vi "Name Bundle Selection.vi"(9 "Current Loop Iteration Even":bool, 10 "Bundler Selections":cluster{string[]}[](array[cluster]), 11 "Node Number":string) -> (2 "Appended Bundler Selections":cluster{string[]}[](array[cluster]))   [LabVIEW 2014, in "Initialization and IO Node Scripting.lvlib"]
uses:
  Initialization and IO Node Scripting.lvlib
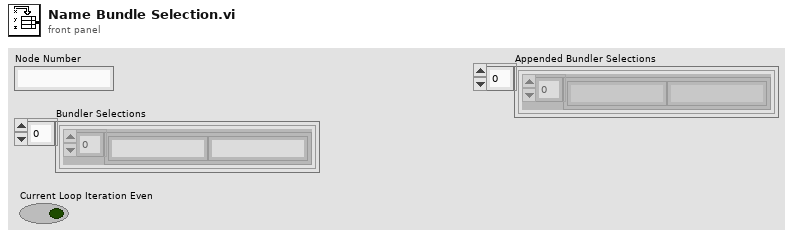
[diagram p1: front panel]
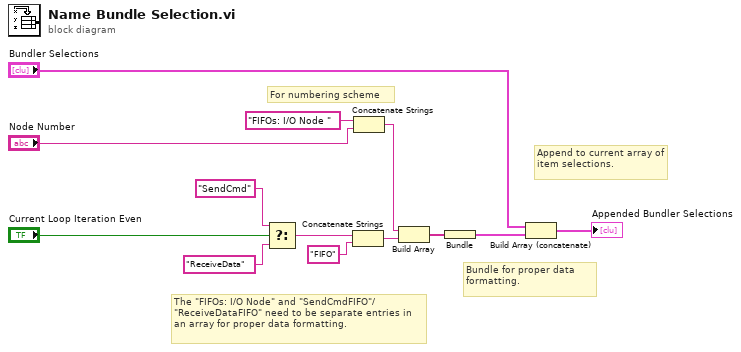
[diagram p0: block diagram]
diagram:
  # "Append to current array of item selections."
  # "Bundle for proper data formatting."
  # "For numbering scheme"
  # "The \"FIFOs: I/O Node\" and \"SendCmdFIFO\"/\"ReceiveDataFIFO\" need to be separate entries in an array for proper data formatting."
  n1 = Select(t="SendCmd" ("string"), s="Current Loop Iteration Even", f="ReceiveData" ("string")) -> (s? t:f=w11:string)
  n2 = Concatenate Strings(w11, "FIFO" ("string")) -> (w13:string)
  n3 = Concatenate Strings("FIFOs: I/O Node " ("string"), "Node Number") -> (w10:string)
  n4 = Build Array(w10, w13) -> (w3:string[])
  n5 = Bundle(w3) -> (w7:cluster{string[]})  [unwired: 1 in]
  n6 = Build Array (concatenate)("Bundler Selections", w7) -> (→"Appended Bundler Selections":cluster{string[]}[])
